vi "Find(End)LoopPair.vi"(9 "Search index":i32, 11 "Mode Array":string[](array[string])) -> (1 "EndLoop index":i32, 2 "Loop index":i32)   [LabVIEW 2013]
doc: "Find matching Loop-EndLoop pair surrounding (inclusive, innermost nesting level) \"Search index\", if it exists. Indices of Loop-EndLoop pair are output. If unpaired Loop or EndLoop is at \"Search index\", the corresponding output mirrors index while the missing pair index is set to -1. Outputs are both -1 if Search index is not within a loop and no un-paired Loop/EndLoop is found."
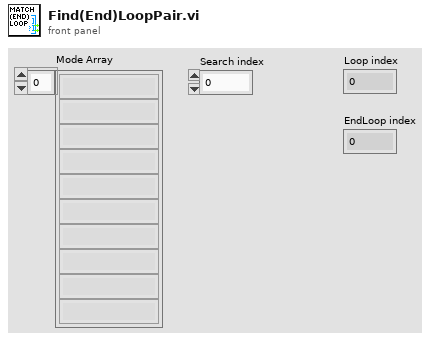
[diagram p1: front panel]
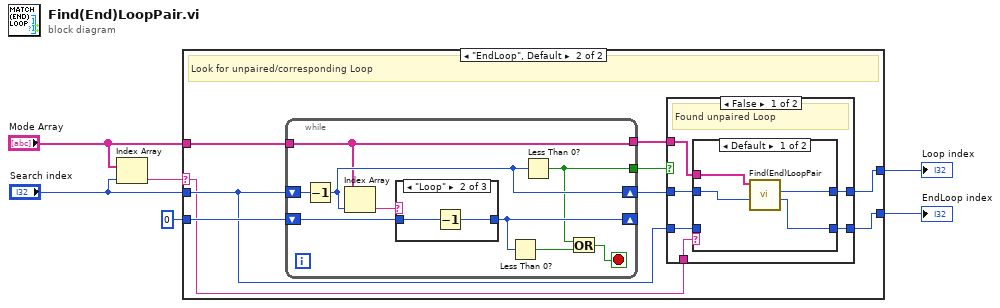
[diagram p0: block diagram]
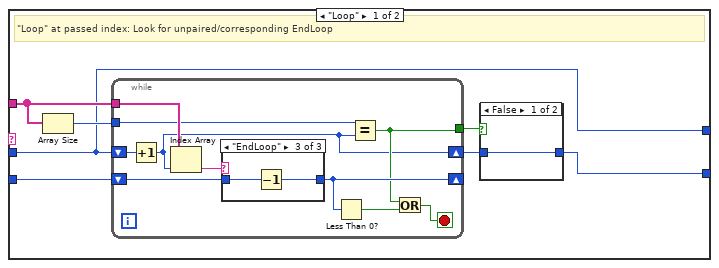
[diagram p2: hidden frame]
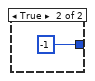
[diagram p3: hidden frame]
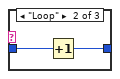
[diagram p5: hidden frame]
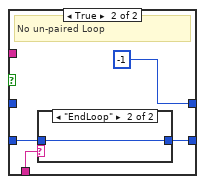
[diagram p7: hidden frame]
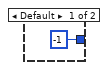
[diagram p8: hidden frame]
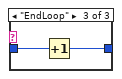
[diagram p10: hidden frame]
diagram:
  n1 = Index Array(array="Mode Array", index="Search index") -> (element=w6:string)
  n2 = case shown="\"EndLoop\", Default" w6 {
    selector: w6 -> [_ w32]
    tunnel: "Mode Array" -> [w13 w39]
    tunnel: "Search index" -> [w10 w34]
    tunnel: [w7 w33] -> w3
    tunnel: 0 ("(End)Loop index") -> [w11 w38]
    tunnel: [w10 w35] -> w2
    frame "Loop" {
      # "\"Loop\" at passed index: Look for unpaired/corresponding EndLoop"
      n3 = Array Size(array=w13) -> (size(s)=w12:i32)
      n4 = while {
        tunnel: w13 -> [w25]
        shift-right: [w22] -> _
        shift-left: w11 -> [w23]
        shift-right: [w16] -> w8
        shift-left: w10 -> [w17]
        tunnel: w12 -> [w21]
        tunnel: [w19] -> w9
        stop <- w18 stop-if-true
        n5 = Increment(x=w17) -> (x+1=w16:i32)
        n6 = Index Array(array=w25, index=w16) -> (element=w24:string)
        n7 = case shown="\"EndLoop\"" w24 {
          tunnel: w23 -> [w26 w28 w30]
          tunnel: [w26 w27 w29] -> w22
          frame Default {
          }
          frame "Loop" {
            n8 = Increment(x=w28) -> (x+1=w27:i32)
          }
          frame "EndLoop" {
            n9 = Decrement(x=w30) -> (x-1=w29:i32)
          }
        }
        n10 = Less Than 0?(x=w22) -> (x < 0?=w20:bool)
        n11 = Equal?(x=w21, y=w16) -> (x = y?=w19:bool)
        n12 = Or(x=w19, y=w20) -> (x .or. y?=w18:bool)
      }
      n13 = case shown="False" w9 {
        tunnel: w8 -> [w14 _]
        tunnel: [w14 -1 ("(End)Loop index")] -> w7
        frame False {
        }
        frame True {
        }
      }
    }
    frame "EndLoop", Default {
      # "Look for unpaired/corresponding Loop"
      n14 = while {
        tunnel: w39 -> [w58]
        shift-right: [w64] -> _
        shift-left: w38 -> [w65]
        shift-right: [w60] -> w36
        shift-left: w34 -> [w61]
        tunnel: [w59] -> w37
        tunnel: [w58] -> w31
        stop <- w62 stop-if-true
        n15 = Decrement(x=w61) -> (x-1=w60:i32)
        n16 = Index Array(array=w58, index=w60) -> (element=w66:string)
        n17 = case shown="\"Loop\"" w66 {
          tunnel: w65 -> [w67 w69 w71]
          tunnel: [w67 w68 w70] -> w64
          frame Default {
          }
          frame "Loop" {
            n18 = Decrement(x=w69) -> (x-1=w68:i32)
          }
          frame "EndLoop" {
            n19 = Increment(x=w71) -> (x+1=w70:i32)
          }
        }
        n20 = Less Than 0?(x=w64) -> (x < 0?=w63:bool)
        n21 = Less Than 0?(x=w60) -> (x < 0?=w59:bool)
        n22 = Or(x=w59, y=w63) -> (x .or. y?=w62:bool)
      }
      n23 = case shown="False" w37 {
        tunnel: w36 -> [w43 _]
        tunnel: [w44 -1 ("(End)Loop index")] -> w35
        tunnel: w34 -> [w41 w52]
        tunnel: [w42 w53] -> w33
        tunnel: w32 -> [w45 w54]
        tunnel: w31 -> [w40 _]
        frame False {
          # "Found unpaired Loop"
          n24 = case shown="Default" w45 {
            tunnel: [w48 w51] -> w44
            tunnel: w43 -> [w49 w51]
            tunnel: [w47 w50] -> w42
            tunnel: w41 -> [_ w50]
            tunnel: w40 -> [w46 _]
            frame Default {
              n25 = call "Find(End)LoopPair.vi"("Search index"=w49, "Mode Array"=w46) -> ("EndLoop index"=w47:i32, "Loop index"=w48:i32)  [unwired: 8 in]
            }
            frame "EndLoop" {
            }
          }
        }
        frame True {
          # "No un-paired Loop"
          n26 = case shown="\"EndLoop\"" w54 {
            tunnel: [-1 ("(End)Loop index") w57] -> w53
            tunnel: w52 -> [_ w57]
            frame Default {
            }
            frame "EndLoop" {
            }
          }
        }
      }
    }
  }
  "Loop index" <- w2
  "EndLoop index" <- w3
